vi "ActuatorFaults.vi"   [LabVIEW 2019]
uses:
  <vilib>/Rock Robotics/WPI/DriverStation/WPI_DriverStationRobotMode2.ctl
  outputs.vi
  dsdata.vi
  refnums.vi
  sensors.vi
  pdpterminals.vi
types:
  T1 = enum16{"DriveControl", "TargetControlH", "FeederStation"}
  T2 = typedef "WPI_DriverStationRobotMode2.ctl" = enum16{"Autonomous Disabled", "Autonomous Enabled", "Teleop Disabled", "Teleop Enabled", "Disconnected", "Finish", "Test Disabled", "Test Enabled", "Emergency Stopped"}
  T3 = typedef "WPI_CompressorDevRef.ctl" = cluster{"DevStatus":errorcluster, "Pneumatics Control Module":u8}
  T4 = typedef "WPI_MotorControlDeviceRef.ctl" = cluster{"DeviceStatus":errorcluster, "Type":T5, "PWM":cluster{"PWM Channel":T6, "DeadBand":T7}, "CAN":cluster{"Device Number":u8, "SetOutput VI Ref":variant, "GetOutput VI Ref":variant, "Enable VI Ref":variant, "Disable VI Ref":variant, "Data":variant}, "Invert":bool, "DIO PWM":cluster{"PWM \"Enable\" Channel":T6, "DIOChannel":T8, "PWM Rate":dbl}}
  T5 = typedef "WPI_MotorControlType.ctl" = enum16{"PWM", "CAN", "DIO PWM"}
  T6 = typedef "FPGA_DIOPWMChannel.ctl" = enum8{"PWM 0", "PWM 1", "PWM 2", "PWM 3", "PWM 4", "PWM 5", "PWM 6", "PWM 7", "PWM 8", "PWM 9", "PWM MXP 0", "PWM MXP 1", "PWM MXP 2", "PWM MXP 3", "PWM MXP 4", "PWM MXP 5", "PWM MXP 6", "PWM MXP 7", "PWM MXP 8", "PWM MXP 9", "Invalid"}
  T7 = typedef "WPI_PWMDeadband.ctl" = cluster{"Name":string, "maxPositivePwm":i32, "minPositivePwm":i32, "centerPwm":i32, "maxNegativePwm":i32, "minNegativePwm":i32, "angularRange":u16}
  T8 = typedef "FPGA_DIOChannel.ctl" = enum8{"DIO 0", "DIO 1", "DIO 2", "DIO 3", "DIO 4", "DIO 5", "DIO 6", "DIO 7", "DIO 8", "DIO 9", "DIO MXP 0", "DIO MXP 1", "DIO MXP 2", "DIO MXP 3", "DIO MXP 4", "DIO MXP 5", "DIO MXP 6", "DIO MXP 7", "DIO MXP 8", "DIO MXP 9", "DIO MXP 10", "DIO MXP 11", "DIO MXP 12", "DIO MXP 13", "DIO MXP 14", "DIO MXP 15", "SPI Port CS1", "SPI Port CS2", "SPI Port CS3", "SPI Port MISO", "SPI Port MOSI", "Invalid"}
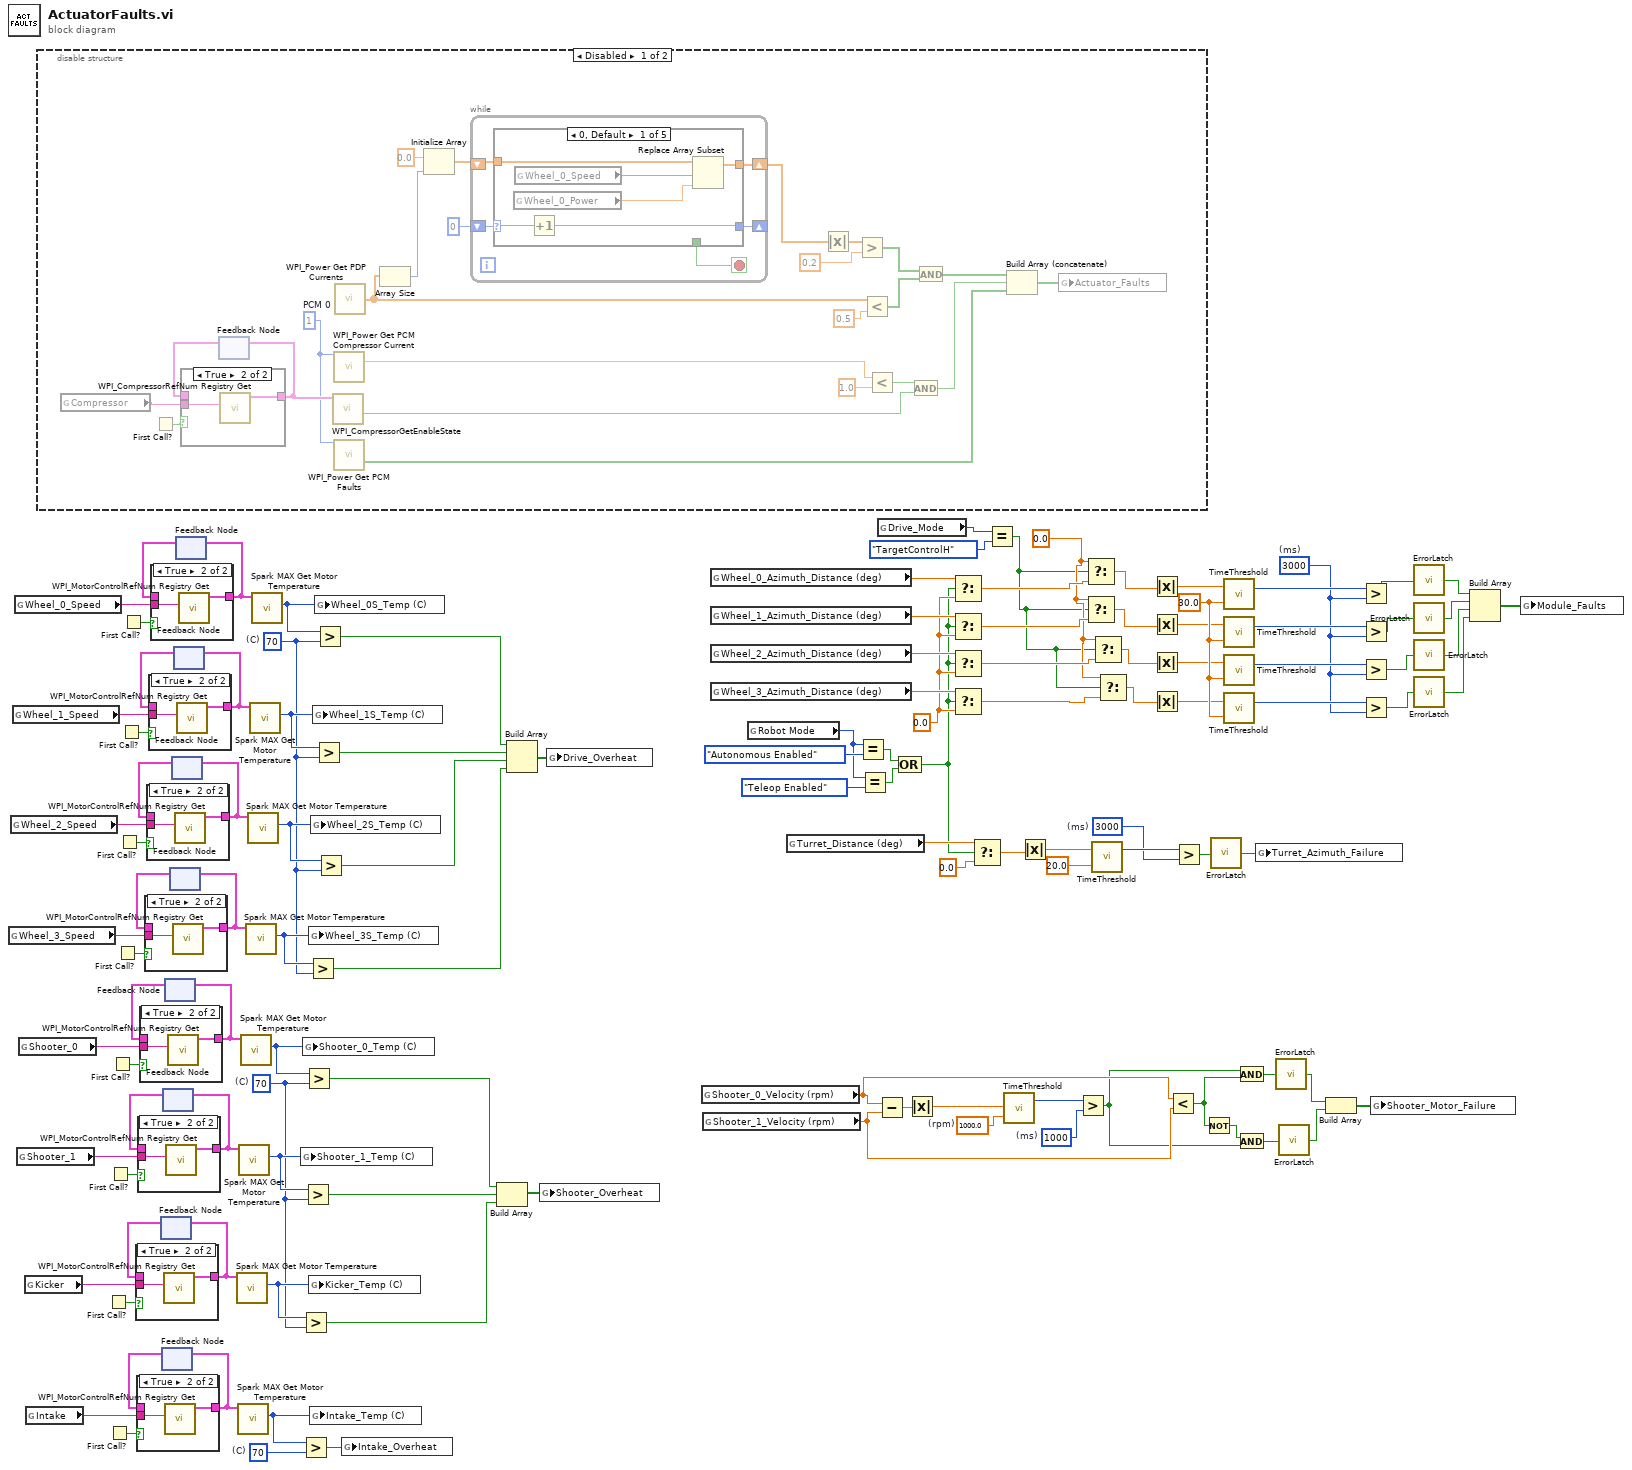
[diagram p0: block diagram]
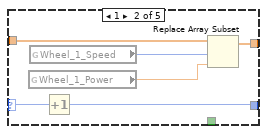
[diagram p10: hidden frame]
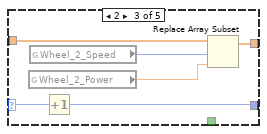
[diagram p11: hidden frame]
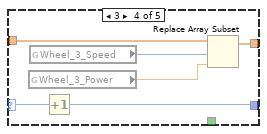
[diagram p12: hidden frame]
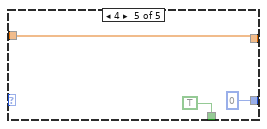
[diagram p13: hidden frame]
diagram:
  w4 = 0.0
  w21 = u32 3000  # (ms)
  w24 = u8 70  # (C)
  w47 = u32 1000  # (ms)
  w49 = 1000.0  # (rpm)
  w31 = u8 70  # (C)
  w65 = 0.0
  w84 = u8 70  # (C)
  w115 = u32 3000  # (ms)
  w114 = 30.0 ("Threshold")
  n1 = global read "refnums.vi" "Wheel_3_Speed"() -> (w90:string)
  n2 = global read "refnums.vi" "Wheel_2_Speed"() -> (w94:string)
  n3 = global read "refnums.vi" "Wheel_1_Speed"() -> (w98:string)
  n4 = global read "refnums.vi" "Wheel_0_Speed"() -> (w102:string)
  n5 = global read "refnums.vi" "Shooter_1"() -> (w58:string)
  n6 = global read "refnums.vi" "Shooter_0"() -> (w62:string)
  n7 = global read "refnums.vi" "Kicker"() -> (w34:string)
  n8 = global read "refnums.vi" "Intake"() -> (w27:string)
  n9 = disable-structure shown="Disabled" {
    frame Disabled {
      w129 = u8 1  # PCM 0
      n10 = global read "refnums.vi" "Compressor"() -> (w128:string)
      n11 = First Call?() -> (First Call?: T/F=w127:bool)
      n12 = feedback #1() -> (w132:T3)  [unwired: 1 in]
      n13 = case shown="True" w127 {
        tunnel: w128 -> [_ w178]
        tunnel: [w176 w177] -> w131
        tunnel: w132 -> [w176 _]
        frame False {
        }
        frame True {
          n14 = call <vilib>:"WPI_CompressorRefNum Registry Get.vi"("refnum name"=w178) -> ("CompressorDevRef"=w177:T3)  [unwired: 9 in, 1 out]
        }
      }
      n15 = feedback-in #1(w131) -> ()
      n16 = call <vilib>:"WPI_CompressorGetEnableState.vi"("CompressorDevRef"=w131) -> ("Compressor Running"=w135:bool)  [unwired: 7 in, 3 out]
      n17 = call <vilib>:"WPI_Power Get PCM Compressor Current.vi"("Pneumatics Control Module (0)"=w129) -> ("current (A)"=w138:dbl)  [unwired: 13 in, 1 out]
      n18 = call <vilib>:"WPI_Power Get PCM Faults.vi"("Pneumatics Control Module (0)"=w129) -> ("All Solenoid Faults"=w130:bool[])  [unwired: 11 in, 3 out]
      n19 = call <vilib>:"WPI_Power Get PDP Currents.vi"() -> ("all currents (A)"=w125:dbl[])  [unwired: 13 in, 2 out]
      n20 = Array Size(array=w125) -> (size(s)=w124:i32)
      n21 = Initialize Array(0.0 ("element"), w124) -> (w121:dbl[])
      n22 = while {
        shift-right: [w146] -> _
        shift-left: 0 -> [w147]
        shift-right: [w144] -> w120
        shift-left: w121 -> [w145]
        stop <- w148 stop-if-true
        n23 = case shown="0, Default" w147 {
          selector: w147 -> [w154 w160 w166 w172 _]
          tunnel: [_ _ _ _ TRUE] -> w148
          tunnel: [w153 w159 w165 w171 0] -> w146
          tunnel: w145 -> [w152 w158 w164 w170 w173]
          tunnel: [w149 w155 w161 w167 w173] -> w144
          frame 0, Default {
            n24 = global read "outputs.vi" "Wheel_0_Power"() -> (w150:dbl)
            n25 = global read "pdpterminals.vi" "Wheel_0_Speed"() -> (w151:i32)
            n26 = Increment(x=w154) -> (x+1=w153:i32)
            n27 = Replace Array Subset(array=w152, new element=w150, index=w151) -> (w149:dbl[])
          }
          frame 1 {
            n28 = global read "outputs.vi" "Wheel_1_Power"() -> (w156:dbl)
            n29 = global read "pdpterminals.vi" "Wheel_1_Speed"() -> (w157:i32)
            n30 = Increment(x=w160) -> (x+1=w159:i32)
            n31 = Replace Array Subset(array=w158, new element=w156, index=w157) -> (w155:dbl[])
          }
          frame 2 {
            n32 = global read "outputs.vi" "Wheel_2_Power"() -> (w162:dbl)
            n33 = global read "pdpterminals.vi" "Wheel_2_Speed"() -> (w163:i32)
            n34 = Increment(x=w166) -> (x+1=w165:i32)
            n35 = Replace Array Subset(array=w164, new element=w162, index=w163) -> (w161:dbl[])
          }
          frame 3 {
            n36 = global read "outputs.vi" "Wheel_3_Power"() -> (w168:dbl)
            n37 = global read "pdpterminals.vi" "Wheel_3_Speed"() -> (w169:i32)
            n38 = Increment(x=w172) -> (x+1=w171:i32)
            n39 = Replace Array Subset(array=w170, new element=w168, index=w169) -> (w167:dbl[])
          }
          frame 4 {
          }
        }
      }
      n40 = Absolute Value(x=w120) -> (abs(x)=w142:dbl[])
      n41 = Greater?(x=w142, y=0.2) -> (0:w140:bool[])
      n42 = Less?(x=w125, y=0.5) -> (x < y?=w139:bool[])
      n43 = Less?(x=w138, y=1.0) -> (x < y?=w136:bool)
      n44 = And(x=w136, y=w135) -> (x .and. y?=w133:bool)
      n45 = And(x=w140, y=w139) -> (x .and. y?=w134:bool[])
      n46 = Build Array (concatenate)(w134, w133, w130) -> (w126:bool[])
      n47 = global write "sensors.vi" "Actuator_Faults"(w126) -> ()
    }
    frame Enabled {
    }
  }
  n48 = First Call?() -> (First Call?: T/F=w36:bool)
  n49 = First Call?() -> (First Call?: T/F=w29:bool)
  n50 = First Call?() -> (First Call?: T/F=w60:bool)
  n51 = First Call?() -> (First Call?: T/F=w64:bool)
  n52 = First Call?() -> (First Call?: T/F=w92:bool)
  n53 = First Call?() -> (First Call?: T/F=w96:bool)
  n54 = First Call?() -> (First Call?: T/F=w100:bool)
  n55 = First Call?() -> (First Call?: T/F=w104:bool)
  n56 = feedback #2() -> (w35:T4)  [unwired: 1 in]
  n57 = case shown="True" w36 {
    tunnel: [w179 w180] -> w33
    tunnel: w35 -> [w179 _]
    tunnel: w34 -> [_ w181]
    frame False {
    }
    frame True {
      n58 = call <vilib>:"WPI_MotorControlRefNum Registry Get.vi"("refnum name"=w181) -> ("MotorControlDevRef"=w180:T4)  [unwired: 9 in, 1 out]
    }
  }
  n59 = feedback-in #2(w33) -> ()
  n60 = feedback #3() -> (w28:T4)  [unwired: 1 in]
  n61 = case shown="True" w29 {
    tunnel: [w182 w183] -> w26
    tunnel: w28 -> [w182 _]
    tunnel: w27 -> [_ w184]
    frame False {
    }
    frame True {
      n62 = call <vilib>:"WPI_MotorControlRefNum Registry Get.vi"("refnum name"=w184) -> ("MotorControlDevRef"=w183:T4)  [unwired: 9 in, 1 out]
    }
  }
  n63 = feedback-in #3(w26) -> ()
  n64 = feedback #4() -> (w59:T4)  [unwired: 1 in]
  n65 = case shown="True" w60 {
    tunnel: [w185 w186] -> w57
    tunnel: w59 -> [w185 _]
    tunnel: w58 -> [_ w187]
    frame False {
    }
    frame True {
      n66 = call <vilib>:"WPI_MotorControlRefNum Registry Get.vi"("refnum name"=w187) -> ("MotorControlDevRef"=w186:T4)  [unwired: 9 in, 1 out]
    }
  }
  n67 = feedback-in #4(w57) -> ()
  n68 = feedback #5() -> (w63:T4)  [unwired: 1 in]
  n69 = case shown="True" w64 {
    tunnel: [w188 w189] -> w61
    tunnel: w63 -> [w188 _]
    tunnel: w62 -> [_ w190]
    frame False {
    }
    frame True {
      n70 = call <vilib>:"WPI_MotorControlRefNum Registry Get.vi"("refnum name"=w190) -> ("MotorControlDevRef"=w189:T4)  [unwired: 9 in, 1 out]
    }
  }
  n71 = feedback-in #5(w61) -> ()
  n72 = feedback #6() -> (w91:T4)  [unwired: 1 in]
  n73 = case shown="True" w92 {
    tunnel: [w191 w192] -> w89
    tunnel: w91 -> [w191 _]
    tunnel: w90 -> [_ w193]
    frame False {
    }
    frame True {
      n74 = call <vilib>:"WPI_MotorControlRefNum Registry Get.vi"("refnum name"=w193) -> ("MotorControlDevRef"=w192:T4)  [unwired: 9 in, 1 out]
    }
  }
  n75 = feedback-in #6(w89) -> ()
  n76 = feedback #7() -> (w95:T4)  [unwired: 1 in]
  n77 = case shown="True" w96 {
    tunnel: [w194 w195] -> w93
    tunnel: w95 -> [w194 _]
    tunnel: w94 -> [_ w196]
    frame False {
    }
    frame True {
      n78 = call <vilib>:"WPI_MotorControlRefNum Registry Get.vi"("refnum name"=w196) -> ("MotorControlDevRef"=w195:T4)  [unwired: 9 in, 1 out]
    }
  }
  n79 = feedback-in #7(w93) -> ()
  n80 = feedback #8() -> (w99:T4)  [unwired: 1 in]
  n81 = case shown="True" w100 {
    tunnel: [w197 w198] -> w97
    tunnel: w99 -> [w197 _]
    tunnel: w98 -> [_ w199]
    frame False {
    }
    frame True {
      n82 = call <vilib>:"WPI_MotorControlRefNum Registry Get.vi"("refnum name"=w199) -> ("MotorControlDevRef"=w198:T4)  [unwired: 9 in, 1 out]
    }
  }
  n83 = feedback-in #8(w97) -> ()
  n84 = feedback #9() -> (w103:T4)  [unwired: 1 in]
  n85 = case shown="True" w104 {
    tunnel: [w200 w201] -> w101
    tunnel: w103 -> [w200 _]
    tunnel: w102 -> [_ w202]
    frame False {
    }
    frame True {
      n86 = call <vilib>:"WPI_MotorControlRefNum Registry Get.vi"("refnum name"=w202) -> ("MotorControlDevRef"=w201:T4)  [unwired: 9 in, 1 out]
    }
  }
  n87 = feedback-in #9(w101) -> ()
  n88 = call <vilib>:"Spark MAX Get Motor Temperature.vi"("MotorControlDevRef in"=w33) -> ("Motor Temperature"=w32:u8)  [unwired: 7 in, 3 out]
  n89 = call <vilib>:"Spark MAX Get Motor Temperature.vi"("MotorControlDevRef in"=w26) -> ("Motor Temperature"=w25:u8)  [unwired: 7 in, 3 out]
  n90 = call <vilib>:"Spark MAX Get Motor Temperature.vi"("MotorControlDevRef in"=w57) -> ("Motor Temperature"=w55:u8)  [unwired: 7 in, 3 out]
  n91 = call <vilib>:"Spark MAX Get Motor Temperature.vi"("MotorControlDevRef in"=w61) -> ("Motor Temperature"=w56:u8)  [unwired: 7 in, 3 out]
  n92 = call <vilib>:"Spark MAX Get Motor Temperature.vi"("MotorControlDevRef in"=w89) -> ("Motor Temperature"=w85:u8)  [unwired: 7 in, 3 out]
  n93 = call <vilib>:"Spark MAX Get Motor Temperature.vi"("MotorControlDevRef in"=w93) -> ("Motor Temperature"=w86:u8)  [unwired: 7 in, 3 out]
  n94 = call <vilib>:"Spark MAX Get Motor Temperature.vi"("MotorControlDevRef in"=w97) -> ("Motor Temperature"=w87:u8)  [unwired: 7 in, 3 out]
  n95 = call <vilib>:"Spark MAX Get Motor Temperature.vi"("MotorControlDevRef in"=w101) -> ("Motor Temperature"=w88:u8)  [unwired: 7 in, 3 out]
  n96 = global write "sensors.vi" "Shooter_1_Temp (C)"(w55) -> ()
  n97 = Greater?(x=w32, y=w31) -> (0:w30:bool)
  n98 = Greater?(x=w25, y=w24) -> (0:w23:bool)
  n99 = global write "sensors.vi" "Shooter_0_Temp (C)"(w56) -> ()
  n100 = Greater?(x=w55, y=w31) -> (0:w53:bool)
  n101 = Greater?(x=w56, y=w31) -> (0:w54:bool)
  n102 = Greater?(x=w85, y=w84) -> (0:w80:bool)
  n103 = global write "sensors.vi" "Wheel_3S_Temp (C)"(w85) -> ()
  n104 = global write "sensors.vi" "Kicker_Temp (C)"(w32) -> ()
  n105 = global write "sensors.vi" "Intake_Temp (C)"(w25) -> ()
  n106 = global write "sensors.vi" "Wheel_2S_Temp (C)"(w86) -> ()
  n107 = global write "sensors.vi" "Wheel_1S_Temp (C)"(w87) -> ()
  n108 = Greater?(x=w87, y=w84) -> (0:w82:bool)
  n109 = global write "sensors.vi" "Wheel_0S_Temp (C)"(w88) -> ()
  n110 = Greater?(x=w88, y=w84) -> (0:w83:bool)
  n111 = Greater?(x=w86, y=w84) -> (0:w81:bool)
  n112 = global write "sensors.vi" "Intake_Overheat"(w23) -> ()
  n113 = Build Array(w54, w53, w30) -> (w52:bool[])
  n114 = Build Array(w83, w82, w81, w80) -> (w79:bool[])
  n115 = global write "sensors.vi" "Shooter_Overheat"(w52) -> ()
  n116 = global write "sensors.vi" "Drive_Overheat"(w79) -> ()
  n117 = global read "sensors.vi" "Shooter_0_Velocity (rpm)"() -> (w46:dbl)
  n118 = global read "sensors.vi" "Shooter_1_Velocity (rpm)"() -> (w45:dbl)
  n119 = global read "outputs.vi" "Wheel_0_Azimuth_Distance (deg)"() -> (w69:dbl)
  n120 = global read "outputs.vi" "Wheel_1_Azimuth_Distance (deg)"() -> (w68:dbl)
  n121 = global read "outputs.vi" "Wheel_2_Azimuth_Distance (deg)"() -> (w67:dbl)
  n122 = global read "outputs.vi" "Wheel_3_Azimuth_Distance (deg)"() -> (w66:dbl)
  n123 = global read "dsdata.vi" "Robot Mode"() -> (w107:T2)
  n124 = global read "outputs.vi" "Turret_Distance (deg)"() -> (w17:dbl)
  n125 = Equal?(x=w107, y=WPI_DriverStationRobotMode2."Autonomous Enabled") -> (x = y?=w106:bool)
  n126 = Equal?(x=w107, y=WPI_DriverStationRobotMode2."Teleop Enabled") -> (x = y?=w105:bool)
  n127 = Subtract(x=w46, y=w45) -> (x-y=w51:dbl)
  n128 = global read "outputs.vi" "Drive_Mode"() -> (w2:T1)
  n129 = Compound Arithmetic op=OR(w106, w105) -> (w16:bool)
  n130 = Absolute Value(x=w51) -> (abs(x)=w50:dbl)
  n131 = Select(t=w69, s=w16, f=w65) -> (s? t:f=w12:dbl)
  n132 = Select(t=w68, s=w16, f=w65) -> (s? t:f=w10:dbl)
  n133 = Select(t=w67, s=w16, f=w65) -> (s? t:f=w8:dbl)
  n134 = Select(t=w66, s=w16, f=w65) -> (s? t:f=w6:dbl)
  n135 = Select(t=w17, s=w16, f=0.0) -> (s? t:f=w18:dbl)
  n136 = Equal?(x=w2, y=T1."TargetControlH" ("Drive_Mode")) -> (x = y?=w1:bool)
  n137 = call "TimeThreshold.vi"("Threshold"=w49, "Current Value"=w50) -> ("Time Above Threshold (ms)"=w48:u32)  [unwired: 1 out]
  n138 = Absolute Value(x=w18) -> (abs(x)=w20:dbl)
  n139 = Greater?(x=w48, y=w47) -> (0:w43:bool)
  n140 = Select(t=w4, s=w1, f=w12) -> (s? t:f=w11:dbl)
  n141 = Select(t=w4, s=w1, f=w10) -> (s? t:f=w9:dbl)
  n142 = call "TimeThreshold.vi"("Threshold"=20.0, "Current Value"=w20) -> ("Time Above Threshold (ms)"=w22:u32)  [unwired: 1 out]
  n143 = Select(t=w4, s=w1, f=w8) -> (s? t:f=w7:dbl)
  n144 = Select(t=w4, s=w1, f=w6) -> (s? t:f=w5:dbl)
  n145 = Absolute Value(x=w11) -> (abs(x)=w113:dbl)
  n146 = Absolute Value(x=w9) -> (abs(x)=w112:dbl)
  n147 = Absolute Value(x=w7) -> (abs(x)=w111:dbl)
  n148 = Absolute Value(x=w5) -> (abs(x)=w110:dbl)
  n149 = Less?(x=w46, y=w45) -> (x < y?=w42:bool)
  n150 = Greater?(x=w22, y=w21) -> (0:w19:bool)
  n151 = Not(x=w42) -> (.not. x?=w44:bool)
  n152 = call "ErrorLatch.vi"("Trigger"=w19) -> ("Latched"=w13:bool)
  n153 = call "TimeThreshold.vi"("Threshold"=w114, "Current Value"=w113) -> ("Time Above Threshold (ms)"=w119:u32)  [unwired: 1 out]
  n154 = call "TimeThreshold.vi"("Threshold"=w114, "Current Value"=w112) -> ("Time Above Threshold (ms)"=w118:u32)  [unwired: 1 out]
  n155 = call "TimeThreshold.vi"("Threshold"=w114, "Current Value"=w111) -> ("Time Above Threshold (ms)"=w117:u32)  [unwired: 1 out]
  n156 = call "TimeThreshold.vi"("Threshold"=w114, "Current Value"=w110) -> ("Time Above Threshold (ms)"=w116:u32)  [unwired: 1 out]
  n157 = And(x=w43, y=w42) -> (x .and. y?=w41:bool)
  n158 = And(x=w44, y=w43) -> (x .and. y?=w40:bool)
  n159 = global write "sensors.vi" "Turret_Azimuth_Failure"(w13) -> ()
  n160 = call "ErrorLatch.vi"("Trigger"=w41) -> ("Latched"=w38:bool)
  n161 = call "ErrorLatch.vi"("Trigger"=w40) -> ("Latched"=w37:bool)
  n162 = Build Array(w38, w37) -> (w39:bool[])
  n163 = Greater?(x=w119, y=w115) -> (0:w73:bool)
  n164 = Greater?(x=w118, y=w115) -> (0:w72:bool)
  n165 = Greater?(x=w117, y=w115) -> (0:w71:bool)
  n166 = Greater?(x=w116, y=w115) -> (0:w70:bool)
  n167 = global write "sensors.vi" "Shooter_Motor_Failure"(w39) -> ()
  n168 = call "ErrorLatch.vi"("Trigger"=w73) -> ("Latched"=w78:bool)
  n169 = call "ErrorLatch.vi"("Trigger"=w72) -> ("Latched"=w77:bool)
  n170 = call "ErrorLatch.vi"("Trigger"=w71) -> ("Latched"=w76:bool)
  n171 = call "ErrorLatch.vi"("Trigger"=w70) -> ("Latched"=w75:bool)
  n172 = Build Array(w78, w77, w76, w75) -> (w74:bool[])
  n173 = global write "sensors.vi" "Module_Faults"(w74) -> ()
